vi "Create One Timeset.vi"(6 "Timeset Name":string="-", 7 "Notes":string, 8 "error in (no error)":errorcluster, 9 "PinStates":T1[](array[typedef]), 10 "OpCode":string, 11 "SPI 3W Pattern Creator in":refnum<class "SPI 3W Pattern Creator.lvclass">) -> (0 "error out":errorcluster, 2 "String  out":string, 3 "SPI 3W Pattern Creator out":refnum<class "SPI 3W Pattern Creator.lvclass">)   [LabVIEW 2018, in "SPI 3W Pattern Creator.lvlib" / "SPI 3W Pattern Creator.lvclass"]
uses:
  SPI 3W Pattern Creator.lvclass
  Interfaces/Protocol Interface.lvlibp/Interfaces/Protocol Interface/Pin State.ctl
  Interfaces/Protocol Interface.lvlibp/Interfaces/Protocol Interface/Protocol Interface.lvclass
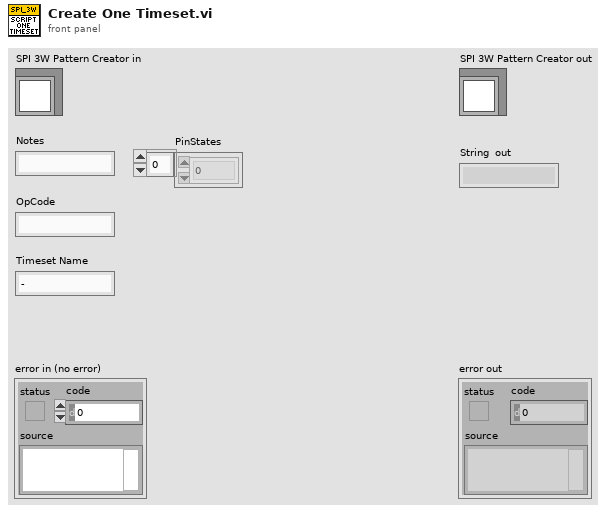
[diagram p1: front panel]
types:
  T1 = typedef "Protocol Interface.lvlibp/Protocol Interface.lvclass/Pin State.ctl" = enum16{"0", "1", "L", "H", "X", "V", "D", "M"}
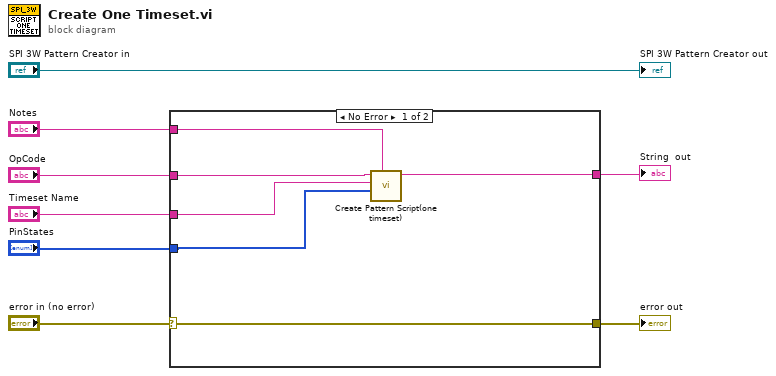
[diagram p0: block diagram]
diagram:
  n1 = case shown="No Error" "error in (no error)" {
    selector: "error in (no error)" -> [w14 w15]
    tunnel: [w14 w15] -> w7
    tunnel: "Notes" -> [w13 _]
    tunnel: "OpCode" -> [w12 _]
    tunnel: "Timeset Name" -> [w11 _]
    tunnel: "PinStates" -> [w10 _]
    tunnel: [w9 _] -> w1
    frame No Error {
      n2 = call "Create Pattern Script(one timeset).vi"("Notes"=w13, "Pin States"=w10, "timeset name"=w11, "opcode"=w12) -> ("string out"=w9:string)  [unwired: 7 in]
    }
    frame Error {
    }
  }
  "error out" <- w7
  "String  out" <- w1
  "SPI 3W Pattern Creator out" <- "SPI 3W Pattern Creator in"
